vi "表达式-顺序等.vi"() -> ()   [LabVIEW 2014]
panel:
  in  "确定按钮":bool
  in  "字符串":string
  in  "组合框":string(combo)
  out "价格 2":dbl
  in  "旋钮 10":i8(knob) scale=0.0..10.0
  out "数值":i32
  in  "旋钮 9":i8(knob) scale=0.0..10.0
  in  "停止":bool
  out "数值 A+B 9":i32
  out "数值 A+B 8":i32
  out "数值 A+B 7":i32
  out "数值 A+B 6":i32
  out "数值 A+B 5":i8
  out "数值A-B 4":i8
  out "数值 A+B 4":i8
  in  "旋钮 4":i8(knob) scale=0.0..10.0
  out "数值A-B 2":i8
  in  "旋钮 2":i8(knob) scale=0.0..10.0
  out "数值 A+B 2":i8
  out "数值x>=5":i8
  in  "表达式2":i8(knob) scale=0.0..10.0
  out "数值x+x*3":i8
  in  "表达式1":i8(knob) scale=0.0..10.0
  in  "减法开关":bool
  in  "加法开关":bool
  out "价格":i32
  in  "选择水果":i32(ring) items=["Orange"=6, "Apple"=3, "Banana"=2]
  in  "旋钮":dbl(knob) scale=0.0..10.0
  out "数值A-B":dbl
  out "数值 A+B":dbl
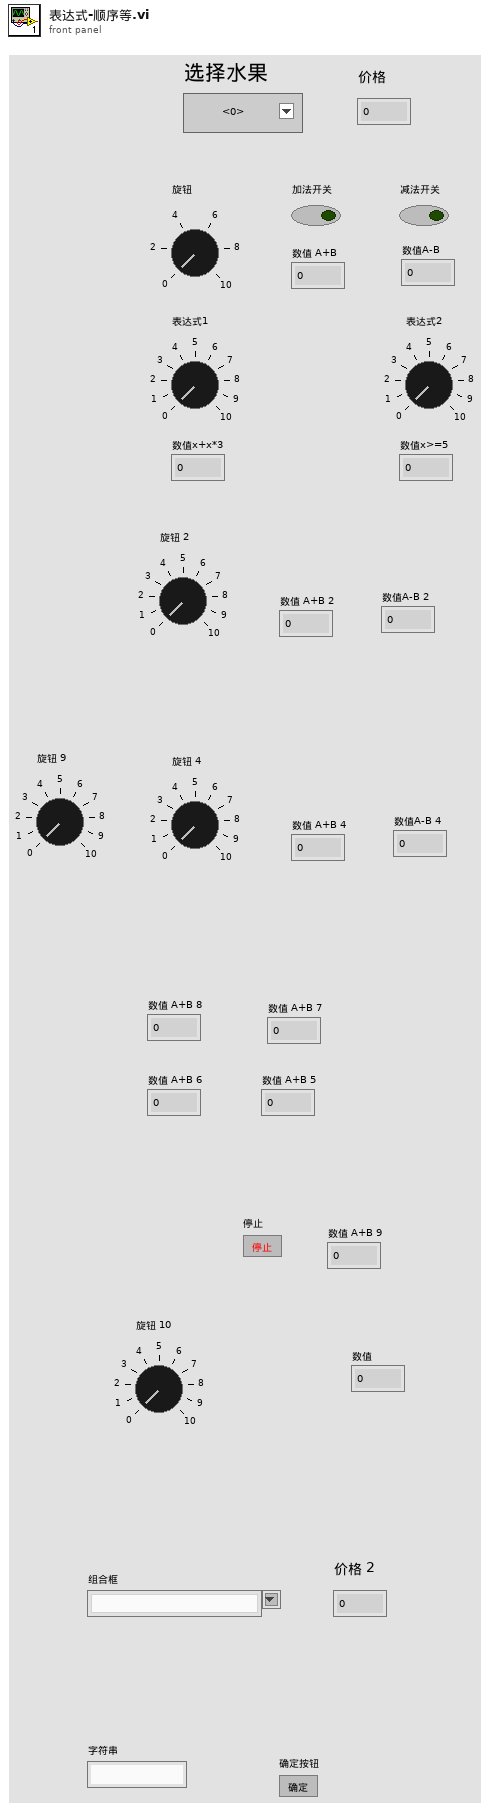
[diagram p1: front panel]
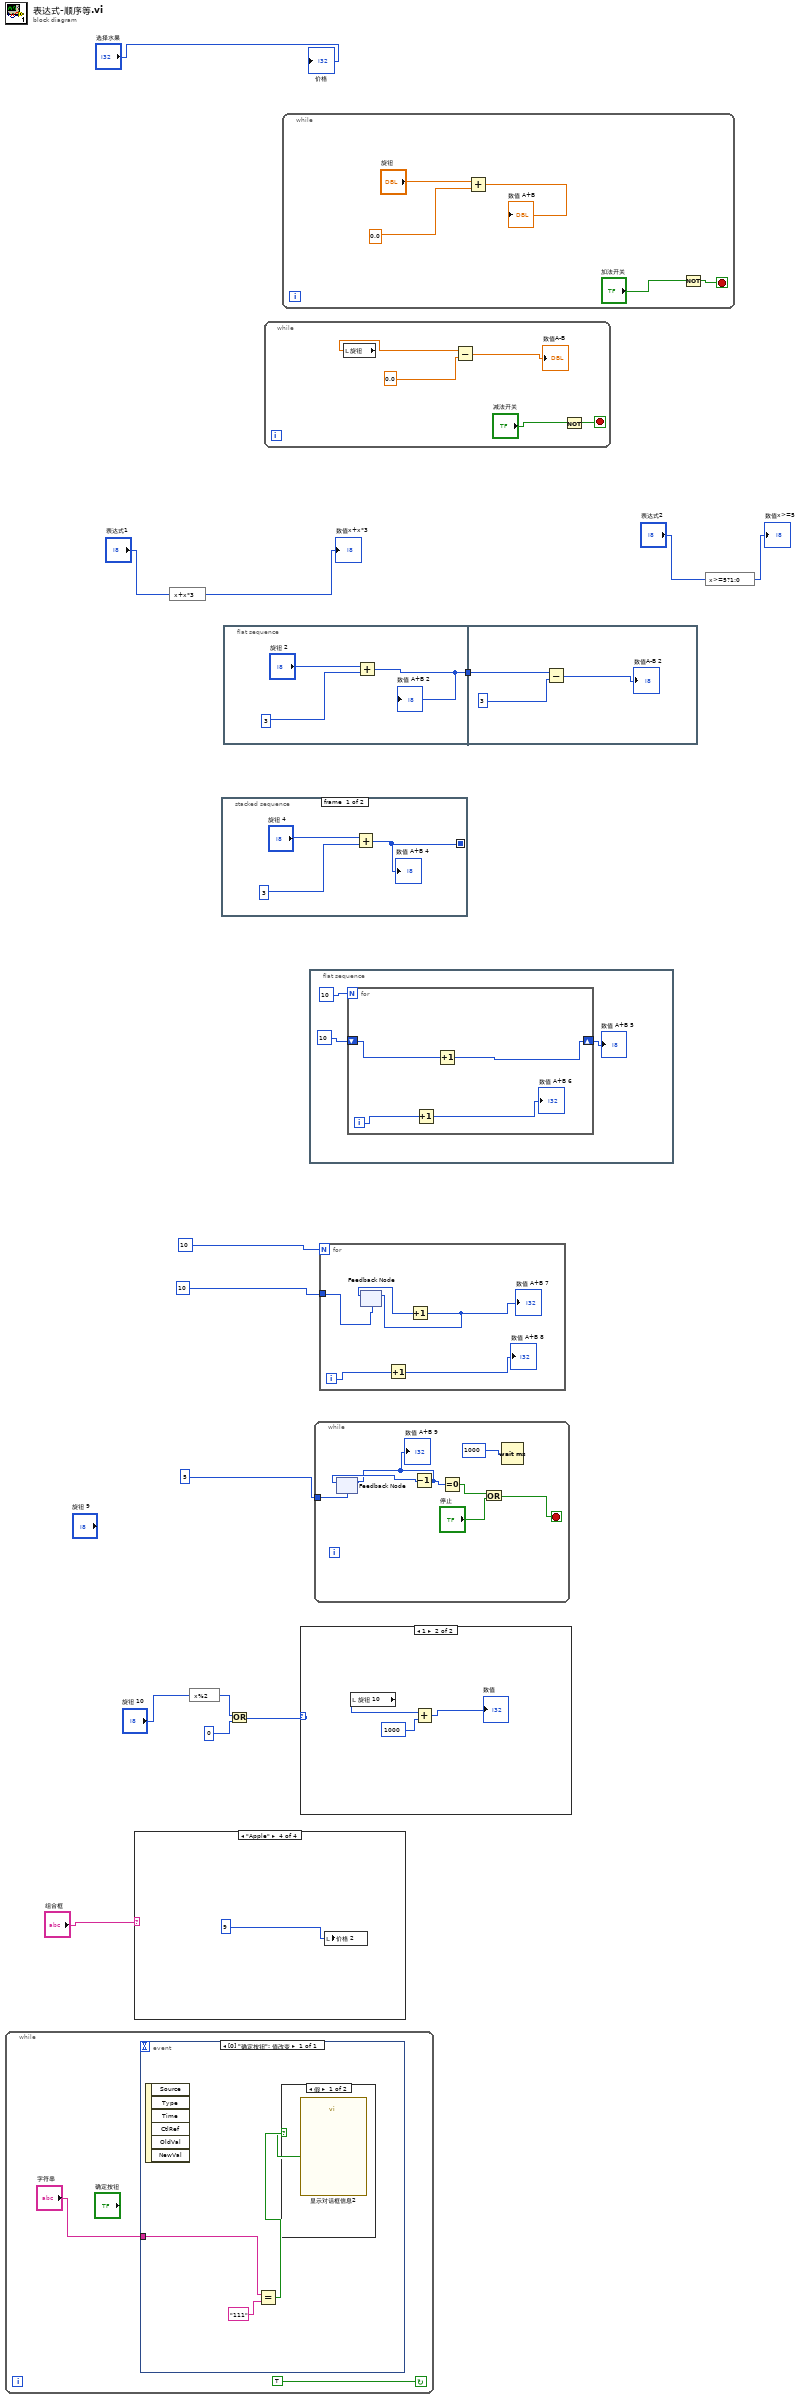
[diagram p0: block diagram]
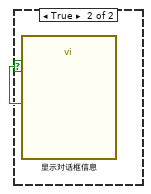
[diagram p2: hidden frame]
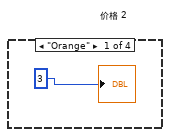
[diagram p3: hidden frame]
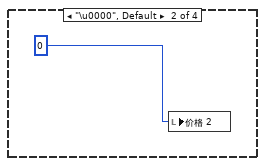
[diagram p4: hidden frame]
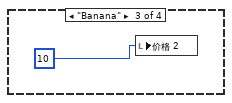
[diagram p5: hidden frame]
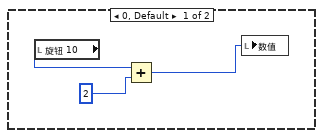
[diagram p6: hidden frame]
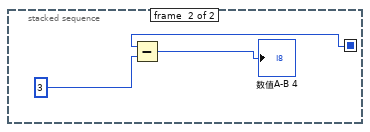
[diagram p7: hidden frame]
diagram:
  n1 = while {
    stop <- TRUE continue-if-true
    n2 = event shown="[0] \"确定按钮\": 值改变" {
      selector: _ -> [_]
      dyn-events: _ -> [_]
      timeout: _ -> [_]
      tunnel: "字符串" -> [w19]
      event "确定按钮": Value Change {
        n3 = event-data() -> ()  [unwired: 1 in, 6 out]
        n4 = Equal?(x=w19, y="111") -> (x = y?=w17:bool)
        n5 = case shown="假" w17 {
          selector: w17 -> [w20 w21]
          frame False {
            n6 = call "显示对话框信息2"("Enable"=w20) -> ()  [unwired: 9 in, 2 out]
          }
          frame True {
            n7 = call "显示对话框信息"("Enable"=w21) -> ()  [unwired: 9 in, 2 out]
          }
        }
      }
    }
  }
  n8 = case shown="\"Apple\"" "组合框" {
    frame "Orange" {
      "价格 2" <- 3
    }
    frame "\u0000", Default {
      n9 = local write "价格 2"(0) -> ()
    }
    frame "Banana" {
      n10 = local write "价格 2"(10) -> ()
    }
    frame "Apple" {
      n11 = local write "价格 2"(9) -> ()
    }
  }
  n12 = expression code="x+x*3"("表达式1") -> (→"数值x+x*3":i8)
  n13 = expression code="x%2"("旋钮 10") -> (w5:i8)
  n14 = stacked-sequence {
    seq-local: [w26 _] -> [_ w29]
    frame #0 {
      n15 = Add(x="旋钮 4", y=i8 3 ("数值")) -> (x+y=w26:i8)
      "数值 A+B 4" <- w26
    }
    frame #1 {
      n16 = Subtract(x=w29, y=i8 3 ("数值")) -> (x-y=→"数值A-B 4":i8)
    }
  }
  n17 = flat-sequence {
    tunnel: [w32] -> w9
    tunnel: w9 -> [w35]
    frame #0 {
      n18 = Add(x="旋钮 2", y=i8 3 ("数值")) -> (x+y=w32:i8)
      "数值 A+B 2" <- w32
    }
    frame #1 {
      n19 = Subtract(x=w35, y=i8 3 ("数值")) -> (x-y=→"数值A-B 2":i8)
    }
  }
  n20 = Or(x=w5, y=0) -> (x .or. y?=w3:i32)
  n21 = while {
    stop <- w39 stop-if-true
    n22 = local read "旋钮"() -> (w40:dbl)
    n23 = Subtract(x=w40, y=0.0 ("数值")) -> (x-y=→"数值A-B":dbl)
    n24 = Not(x="减法开关") -> (.not. x?=w39:bool)
  }
  n25 = while {
    stop <- w44 stop-if-true
    n26 = Add(x="旋钮", y=0.0 ("数值")) -> (x+y=→"数值 A+B":dbl)
    n27 = Not(x="加法开关") -> (.not. x?=w44:bool)
  }
  n28 = case shown="1" w3 {
    frame 0, Default {
      n29 = local read "旋钮 10"() -> (w50:i8)
      n30 = Add(x=w50, y=2) -> (x+y=w48:i32)
      n31 = local write "数值"(w48) -> ()
    }
    frame 1 {
      n32 = local read "旋钮 10"() -> (w51:i8)
      n33 = Add(x=w51, y=1000) -> (x+y=→"数值":i32)
    }
  }
  n34 = flat-sequence {
    frame #0 {
      n35 = for {
        N: 10 -> [_]
        shift-right: [w59] -> w55
        shift-left: 10 -> [w58]
        i -> [w60]
        n36 = Increment(x=w60) -> (x+1=→"数值 A+B 6":i32)
        n37 = Increment(x=w58) -> (x+1=w59:i32)
      }
      "数值 A+B 5" <- w55
    }
  }
  n38 = while {
    tunnel: u8 5 -> [w66]
    stop <- w63 stop-if-true
    n39 = feedback #1(w66) -> (w65:u8)
    n40 = Decrement(x=w65) -> (x-1=w62:u8)
    "数值 A+B 9" <- w62
    n41 = feedback-in #1(w62) -> ()
    n42 = Equal To 0?(x=w62) -> (x = 0?=w61:bool)
    n43 = Or(x=w61, y="停止") -> (x .or. y?=w63:bool)
    n44 = Wait (ms)(milliseconds to wait=1000) -> ()  [unwired: 1 out]
  }
  n45 = for {
    N: 10 -> [_]
    tunnel: 10 -> [w68]
    i -> [w72]
    n46 = feedback #2(w68) -> (w70:i32)
    n47 = Increment(x=w72) -> (x+1=→"数值 A+B 8":i32)
    n48 = Increment(x=w70) -> (x+1=w69:i32)
    "数值 A+B 7" <- w69
    n49 = feedback-in #2(w69) -> ()
  }
  n50 = expression code="x>=5?1:0"("表达式2") -> (→"数值x>=5":i8)
  "价格" <- "选择水果"
